vi "Append User ID To Section Label.vi"(0 "VI reference":refnum<vi>, 5 "Path (dialog)":path=path "C:/ProgramData/EPL/CFTS Defaults.ini", 7 "User":string, 9 "Section must exist?":bool, 11 "error in (no error)":errorcluster) -> (4 "VI reference (thru)":refnum<vi>, 6 "Path (thru)":path, 8 "Section Name":string, 15 "error out":errorcluster)   [LabVIEW 2020]
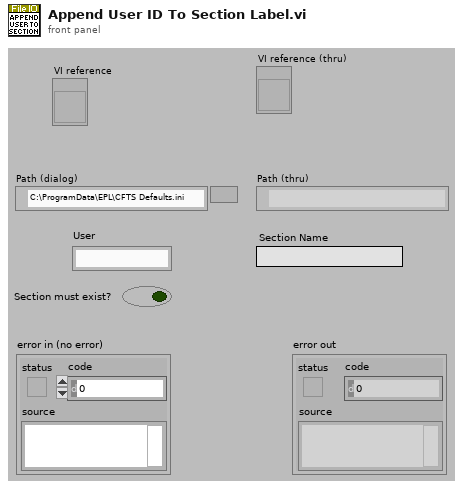
[diagram p1: front panel]
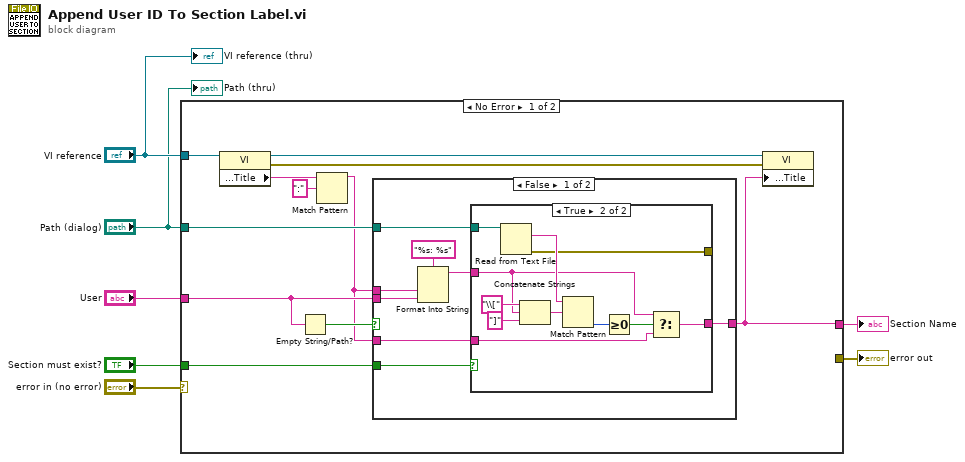
[diagram p0: block diagram]
diagram:
  n1 = case shown="No Error" "error in (no error)" {
    selector: "error in (no error)" -> [_ w40]
    tunnel: [_ w40] -> w6
    tunnel: "VI reference" -> [w17 _]
    tunnel: "User" -> [w16 _]
    tunnel: "Section must exist?" -> [w12 _]
    tunnel: "Path (dialog)" -> [w11 _]
    tunnel: [w10 _] -> w1
    frame No Error {
      n2 = property class="VI"(reference=w17) -> (reference out=w13:refnum<vi>, error out=w8:errorcluster, "Front Panel.Title"=w15:string)  [unwired: 1 in]
      n3 = Empty String/Path?(string/path=w16) -> (empty?=w18:bool)
      n4 = Match Pattern(string=w15, regular expression=":") -> (before substring=w9:string)  [unwired: 1 in, 3 out]
      n5 = case shown="False" w18 {
        tunnel: w9 -> [w25 w39]
        tunnel: [w20 w39] -> w10
        tunnel: w16 -> [w24 _]
        tunnel: w12 -> [w22 _]
        tunnel: w11 -> [w21 _]
        tunnel: w9 -> [w19 _]
        frame False {
          n6 = Format Into String(format string="%s: %s", w25, w24) -> (resulting string=w23:string)  [unwired: 2 in, 1 out]
          n7 = case shown="True" w22 {
            tunnel: w23 -> [w27 w31]
            tunnel: w21 -> [_ w38]
            tunnel: [w27 w30] -> w20
            tunnel: w19 -> [_ w29]
            tunnel: [_ w28] -> _
            frame False {
            }
            frame True {
              n8 = Read from Text File(file (use dialog)=w38) -> (text=w34:string, error out=w28:errorcluster)  [unwired: 3 in, 2 out]
              n9 = Concatenate Strings("\\[" ("string"), w31, "]" ("string")) -> (w37:string)
              n10 = Match Pattern(string=w34, regular expression=w37) -> (offset past match=w33:i32)  [unwired: 1 in, 3 out]
              n11 = Greater Or Equal To 0?(x=w33) -> (x >= 0?=w32:bool)
              n12 = Select(t=w31, s=w32, f=w29) -> (s? t:f=w30:string)
            }
          }
        }
        frame True {
        }
      }
      n13 = property class="VI"(reference=w13, error in=w8, "Front Panel.Title"=w10) -> ()  [unwired: 2 out]
    }
    frame Error {
    }
  }
  "error out" <- w6
  "Section Name" <- w1
  "VI reference (thru)" <- "VI reference"
  "Path (thru)" <- "Path (dialog)"
